vi "Scatter1000.vi"   [LabVIEW 2013]
uses:
  <vilib>/Heliosphere Research LLC/Advanced Plotting Toolkit/Advanced Plotting Toolkit.lvlib
types:
  T1 = typedef "Advanced Plotting Toolkit.lvlib/PlotID.ctl" = i32
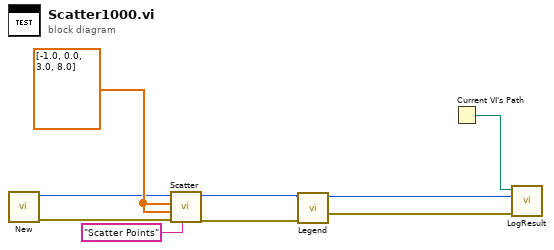
[diagram p0: block diagram]
diagram:
  w8 = dbl[] [-1.0, 0.0, 3.0, 8.0] ("X Data")
  n1 = call <vilib>:"New.vi"() -> ("error out"=w6:errorcluster, "Plot ID"=w7:T1)  [unwired: 10 in]
  n2 = call <vilib>:"Scatter.vi"("Legend Title"="Scatter Points", "error in (no error)"=w6, "Y Data"=w8, "X Data"=w8, "Plot ID"=w7) -> ("error out"=w1:errorcluster, "Plot ID Out"=w4:T1)  [unwired: 5 in]
  n3 = call <vilib>:"Legend.vi"("error in (no error)"=w1, "Plot ID"=w4) -> ("error out"=w2:errorcluster, "Plot ID Out"=w3:T1)  [unwired: 8 in]
  n4 = Current VI's Path() -> (path=w9:path)
  n5 = call "LogResult.vi"("Test Result"=w2, "Test Artifact"=w3, "VI Path"=w9) -> ()  [unwired: 9 in]
